vi "3D Single Mouse Movie.vi"() -> ()   [LabVIEW 2011]
uses:
  <vilib>/vision/NI_Vision_Development_Module.lvlib
panel:
  out "Waveform Graph":dbl[](graph)
  in  "Maximum height 2":i32=64
  in  "Direction (NW) 2":T1(ring)
  in  "3D options 2":T2={"alpha"=30.0, "beta"=30.0, "border"=20, "background"=85, "plane"=2} {"beta" min=15 max=45 format="%.2f"; "alpha" min=15 max=45 format="%.2f"}
  in  "3D options":T2={"alpha"=30.0, "beta"=30.0, "border"=20, "background"=85, "plane"=2} {"beta" min=15 max=45 format="%.2f"; "alpha" min=15 max=45 format="%.2f"}
  in  "Direction (NW)":T1(ring)
  in  "Maximum height":i32=64
  in  "Size reduction":i32=2
  out "Image 2":T3(plugin-control)
  out "Just Mouse":T3(plugin-control)
  out "Image #":i32
  out "Image":T3(plugin-control)
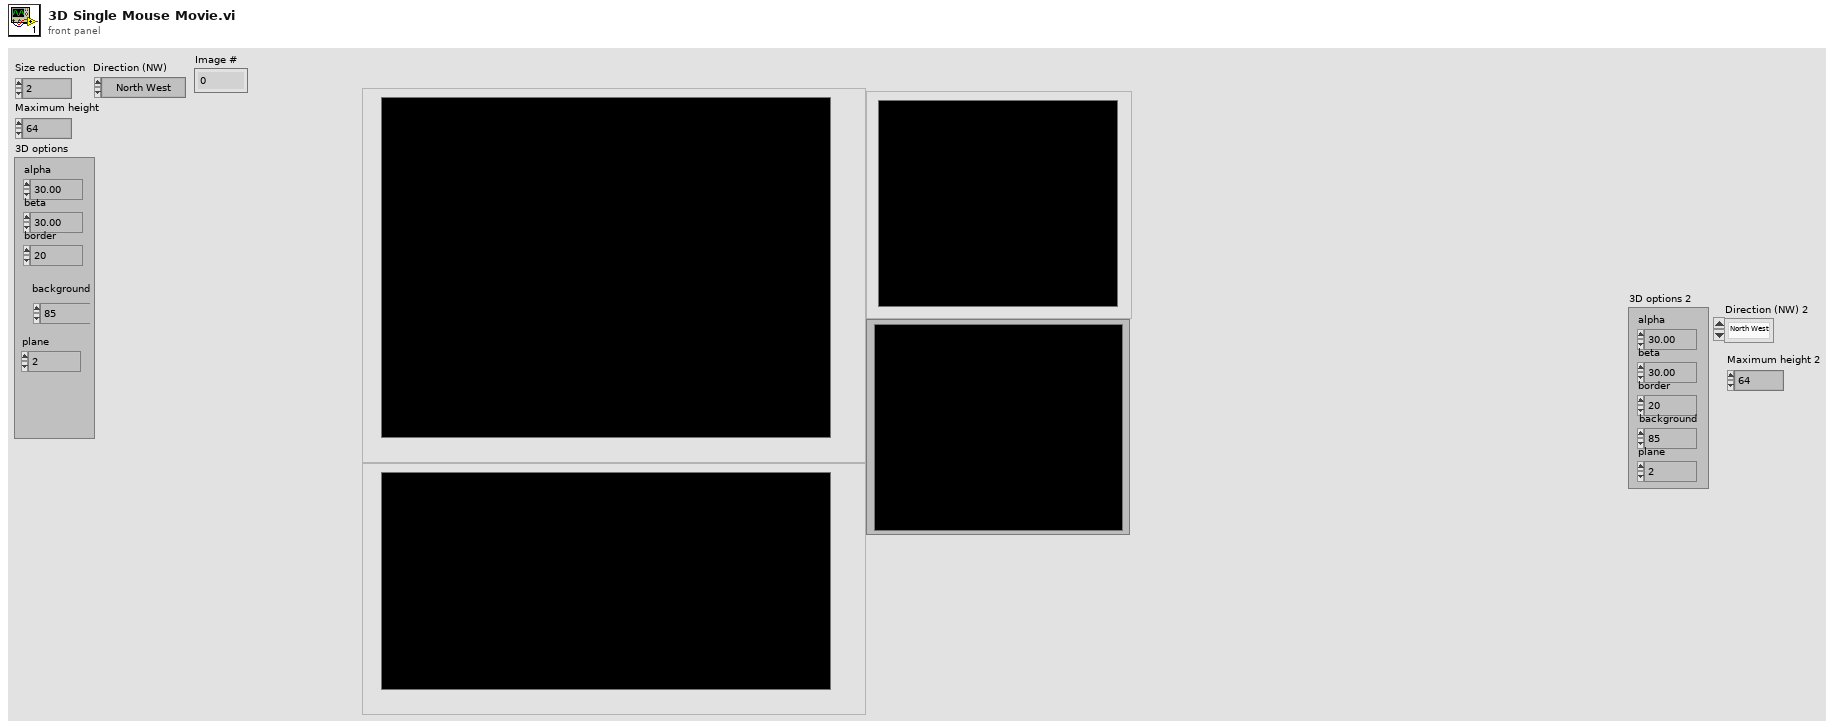
[diagram p1: front panel]
types:
  T1 = enum32{"North West", "South West", "South East", "North East"}
  T2 = cluster{"alpha":sgl, "beta":sgl, "border":i32, "background":i32, "plane":i32}
  T3 = typedef "IMAQ Image.ctl" = refnum<image>
  T4 = typedef "Image Type" = u32
  T5 = cluster{"X Size":i32, "Y Size":i32, "% Tolerance":i32}
  T6 = cluster{"Area":dbl, "Number of Holes":dbl, "Bounding Rect":cluster{"Left":dbl, "Top":dbl, "Right":dbl, "Bottom":dbl}, "Center of Mass":cluster{"X":dbl, "Y":dbl}, "Orientation":dbl, "Dimensions":cluster{"Width":dbl, "Height":dbl}}[]
  T7 = cluster{"Area":dbl, "Number of Holes":dbl, "Bounding Rect":cluster{"Left":dbl, "Top":dbl, "Right":dbl, "Bottom":dbl}, "Center of Mass":cluster{"X":dbl, "Y":dbl}, "Orientation":dbl, "Dimensions":cluster{"Width":dbl, "Height":dbl}}
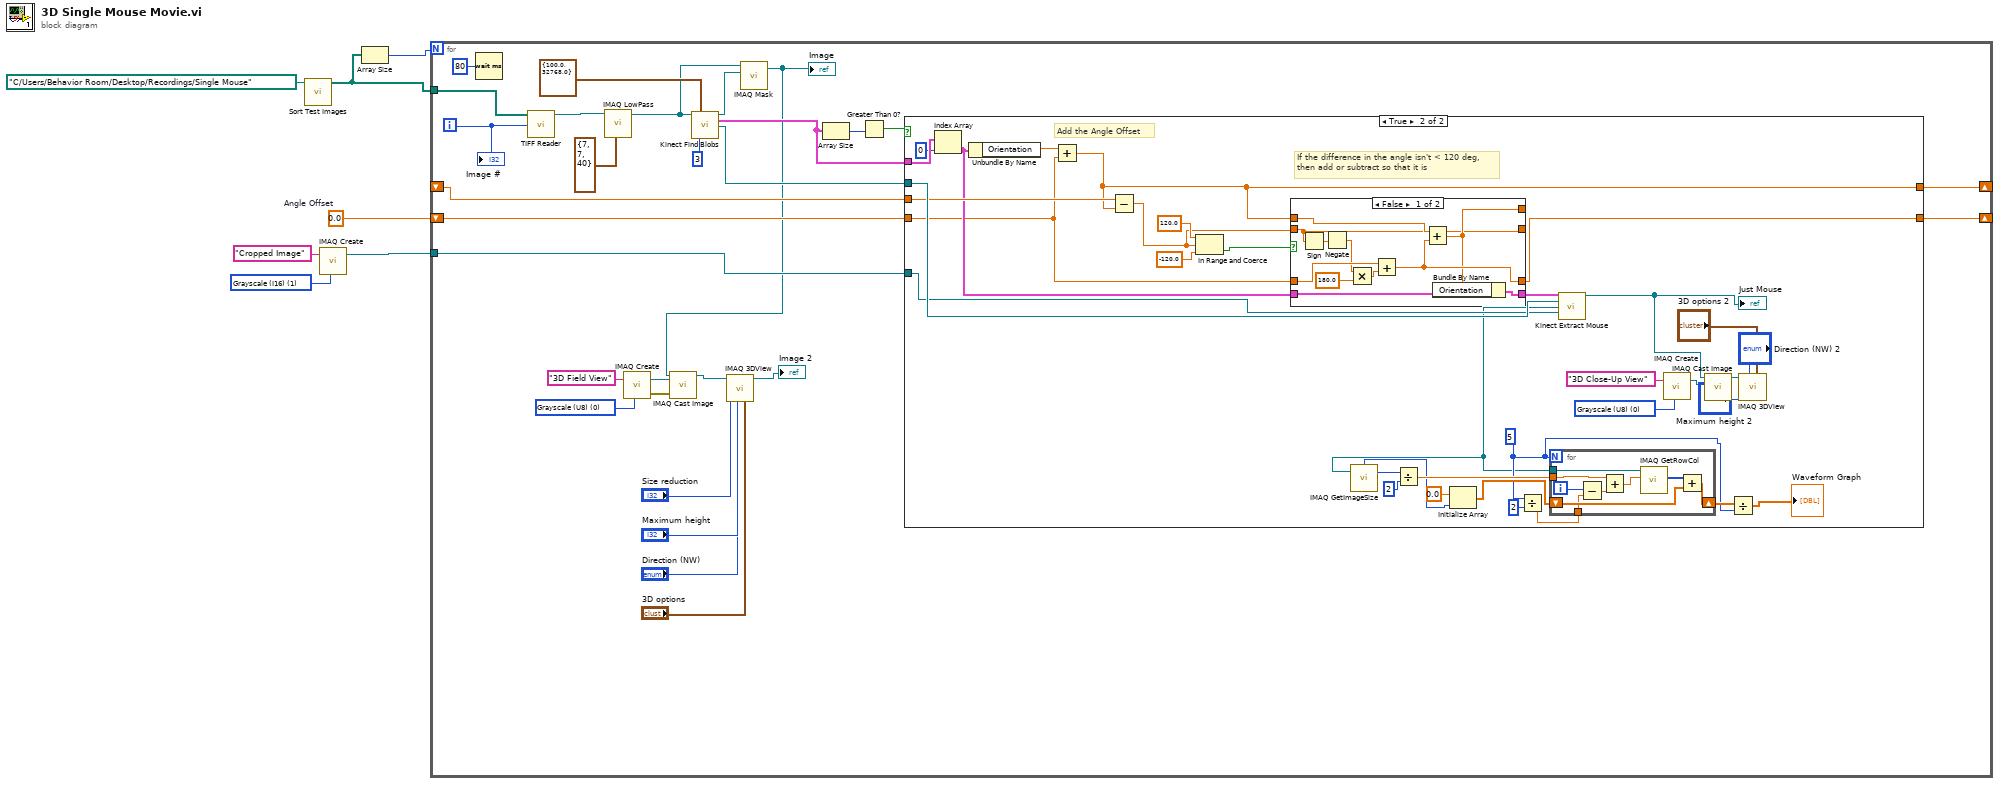
[diagram p0: block diagram]
diagram:
  w2 = 0.0  # Angle Offset
  w4 = T4 1 items=["Grayscale (U8)", "Grayscale (I16)", "Grayscale (SGL)", "Complex (CSG)", "RGB (U32)", "HSL (U32)", "RGB (U64)", "Grayscale (U16)"] ("Image Type")
  n1 = call "Sort Test Images.vi"("path"=path "C:/Users/Behavior Room/Desktop/Recordings/Single Mouse") -> ("Array"=w6:path[])  [unwired: 10 in]
  n2 = call "IMAQ Create"("Image Name"="Cropped Image", "Image Type"=w4) -> ("New Image"=w3:T3)  [unwired: 3 in, 1 out]
  n3 = Array Size(array=w6) -> (size(s)=w7:i32)
  n4 = for {
    N: w7 -> [_]
    tunnel: w6 -> [w36]
    tunnel: w3 -> [w29]
    shift-right: [w26] -> _
    shift-left: _ -> [w25]
    shift-right: [w23] -> _
    shift-left: w2 -> [w24]
    i -> [w35]
    w18 = T4 0 items=["Grayscale (U8)", "Grayscale (I16)", "Grayscale (SGL)", "Complex (CSG)", "RGB (U32)", "HSL (U32)", "RGB (U64)", "Grayscale (U16)"] ("Image Type")
    n5 = Wait (ms)(milliseconds to wait=u32 80) -> ()  [unwired: 1 out]
    n6 = call "TIFF Reader.vi"("index"=w35, "Array"=w36) -> ("Image Out"=w21:T3)  [unwired: 9 in]
    n7 = call "IMAQ LowPass"("Image Src"=w21, "Size & Tolerance"=T5 {"X Size"=7, "Y Size"=7, "% Tolerance"=40}) -> ("Image Dst Out"=w15:T3)  [unwired: 5 in, 1 out]
    n8 = call "IMAQ Create"("Image Name"="3D Field View", "Image Type"=w18) -> ("New Image"=w16:T3, "error out"=w17:errorcluster)  [unwired: 3 in]
    n9 = call "Kinect Find Blobs.vi"("Image Src"=w15, "Range"=cluster{"Lower value":sgl, "Upper value":sgl} {"Lower value"=100.0, "Upper value"=32768.0}, "Number of Erosion"=3) -> ("Masked Image Out"=w27:T3, "Particle Reports (Pixels)"=w30:T6, "Src Image Out"=w28:T3)  [unwired: 10 in]
    n10 = call "IMAQ Mask"("Image Mask"=w27, "Image Src"=w15) -> ("Image Dst Out"=w8:T3)  [unwired: 3 in, 1 out]
    "Image" <- w8
    n11 = call "IMAQ Cast Image"("error in (no error)"=w17, "Image Dst"=w16, "Image Src"=w8) -> ("Image Dst Out"=w14:T3)  [unwired: 7 in, 1 out]
    n12 = call "IMAQ 3DView"("3D options"="3D options", "Maximum height"="Maximum height", "Direction (NW)"="Direction (NW)", "Size reduction"="Size reduction", "Image Src"=w14) -> ("Image Dst Out"=→"Image 2":T3)  [unwired: 5 in, 1 out]
    n13 = Array Size(array=w30) -> (size(s)=w32:i32)
    n14 = Greater Than 0?(x=w32) -> (x > 0?=w31:bool)
    n15 = case shown="True" w31 {
      tunnel: w30 -> [_ w72]
      tunnel: w28 -> [_ w70]
      tunnel: w29 -> [_ w69]
      tunnel: [w38 w58] -> w26
      tunnel: w25 -> [w38 w68]
      tunnel: w24 -> [w37 w60]
      tunnel: [w37 w59] -> w23
      frame False {
      }
      frame True {
        w46 = T4 0 items=["Grayscale (U8)", "Grayscale (I16)", "Grayscale (SGL)", "Complex (CSG)", "RGB (U32)", "HSL (U32)", "RGB (U64)", "Grayscale (U16)"] ("Image Type")
        w48 = 5
        # "If the difference in the angle isn't < 120 deg,\nthen add or subtract so that it is"
        # "Add the Angle Offset"
        n16 = Index Array(array=w72, index=0) -> (element=w63:T7)
        n17 = Unbundle By Name(w63) -> ("Orientation"=w64:dbl)
        n18 = Add(x=w64, y=w60) -> (x+y=w58:dbl)
        n19 = Subtract(x=w68, y=w58) -> (x-y=w61:dbl)
        n20 = In Range and Coerce(upper limit=120.0, x=w61, lower limit=-120.0 ("upper limit")) -> (In Range?=w65:bool)  [unwired: 1 out]
        n21 = case shown="False" w65 {
          tunnel: w63 -> [w89 w96]
          tunnel: [w88 w96] -> w62
          tunnel: w61 -> [w82 w93]
          tunnel: [w90 w95] -> w59
          tunnel: w60 -> [w92 w95]
          tunnel: w58 -> [w91 w94]
          tunnel: [w83 w94] -> _
          tunnel: [w82 w93] -> _
          frame False {
            n22 = Sign(1:w82) -> (0:w87:dbl)
            n23 = Negate(x=w87) -> (-x=w86:dbl)
            n24 = Multiply(x=w86, y=180.0) -> (x*y=w85:dbl)
            n25 = Add(x=w92, y=w85) -> (x+y=w90:dbl)
            n26 = Add(x=w91, y=w90) -> (x+y=w83:dbl)
            n27 = Bundle By Name(cluster=w89, "Orientation"=w83) -> (w88:T7)
          }
          frame True {
          }
        }
        n28 = Divide(x=w48, y=2) -> (x/y=w53:dbl)
        n29 = call "Kinect Extract Mouse.vi"("Particle Report"=w62, "Image Src"=w70, "Image Dst"=w69) -> ("Cropped Image Out"=w44:T3)  [unwired: 11 in, 1 out]
        "Just Mouse" <- w44
        n30 = call "IMAQ GetImageSize"("Image"=w44) -> ("Y Resolution"=w57:i32, "X Resolution"=w51:i32)  [unwired: 3 in, 1 out]
        n31 = Divide(x=w57, y=2) -> (x/y=w55:dbl)
        n32 = Initialize Array(0.0 ("element"), w51) -> (w50:dbl[])
        n33 = for {
          N: w48 -> [_]
          tunnel: w44 -> [w81]
          tunnel: w55 -> [w77]
          shift-right: [w79] -> w49
          shift-left: w50 -> [w78]
          tunnel: w53 -> [w73]
          i -> [w75]
          n34 = Subtract(x=w75, y=w73) -> (x-y=w74:dbl)
          n35 = Add(x=w77, y=w74) -> (x+y=w76:dbl)
          n36 = call "IMAQ GetRowCol"("Image"=w81, "Number"=w76) -> ("Pixels (I16)"=w80:i16[])  [unwired: 4 in, 4 out]
          n37 = Add(x=w80, y=w78) -> (x+y=w79:dbl[])
        }
        n38 = call "IMAQ Create"("Image Name"="3D Close-Up View", "Image Type"=w46) -> ("New Image"=w45:T3)  [unwired: 3 in, 1 out]
        n39 = call "IMAQ Cast Image"("Image Dst"=w45, "Image Src"=w44) -> ("Image Dst Out"=w43:T3)  [unwired: 8 in, 1 out]
        n40 = Divide(x=w49, y=w48) -> (x/y=→"Waveform Graph":dbl[])
        n41 = call "IMAQ 3DView"("3D options"="3D options 2", "Maximum height"="Maximum height 2", "Direction (NW)"="Direction (NW) 2", "Image Src"=w43) -> ()  [unwired: 6 in, 2 out]
      }
    }
    "Image #" <- w35
  }
